vi "Controller Orbit Correction Algorithm.vi"(6 "Resest?":bool, 8 "error in (no error)":errorcluster, 9 "Initial Corrector Kick Vector":dbl[](array[numeric]), 10 "Beam Position Vector":dbl[](array[numeric]), 11 "FOFB Variables":T1) -> (0 "error out":errorcluster, 2 "Corrector Kick Vector":dbl[](array[numeric]), 3 "Good value?":bool=TRUE)   [LabVIEW 2011, in "Controller VIs.lvlib"]
doc: "Computes the correction algorithm to the selected BPM readings and returns the calculated corrector kick vector to be applied to the FOFB actuators."
uses:
  Controller VIs.lvlib
  Types Definitions/Type FOFB Variables.ctl
  Common VIs.lvlib
  Type Definitions.lvlib
panel:
  in  "Maximum allowed disturbance (mm) (1.5)":dbl=1.5 format="%#_6f"
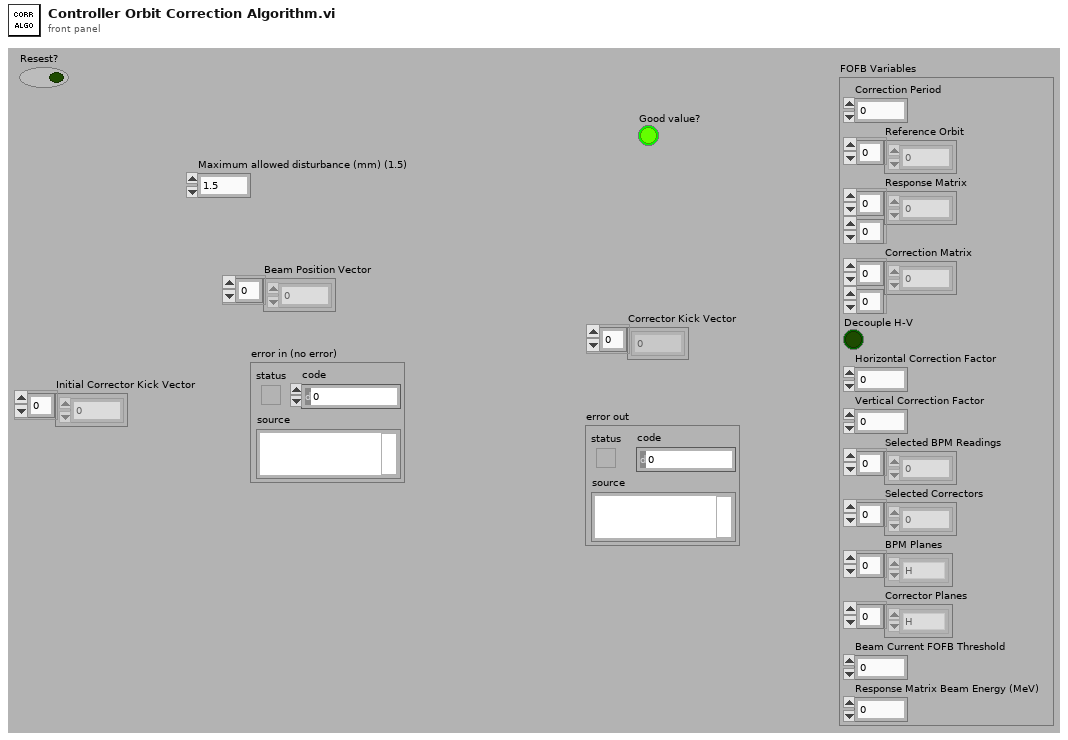
[diagram p1: front panel]
types:
  T1 = typedef "Type Definitions.lvlib/Type FOFB Variables.ctl" = cluster{"Correction Period":u32, "Reference Orbit":dbl[], "Response Matrix":dbl[][], "Correction Matrix":dbl[][], "Decouple H-V":bool, "Horizontal Correction Factor":dbl, "Vertical Correction Factor":dbl, "Selected BPM Readings":u32[], "Selected Correctors":u32[], "BPM Planes":enum8{"H", "V"}[], "Corrector Planes":enum8{"H", "V"}[], "Beam Current FOFB Threshold":dbl, "Response Matrix Beam Energy (MeV)":dbl}
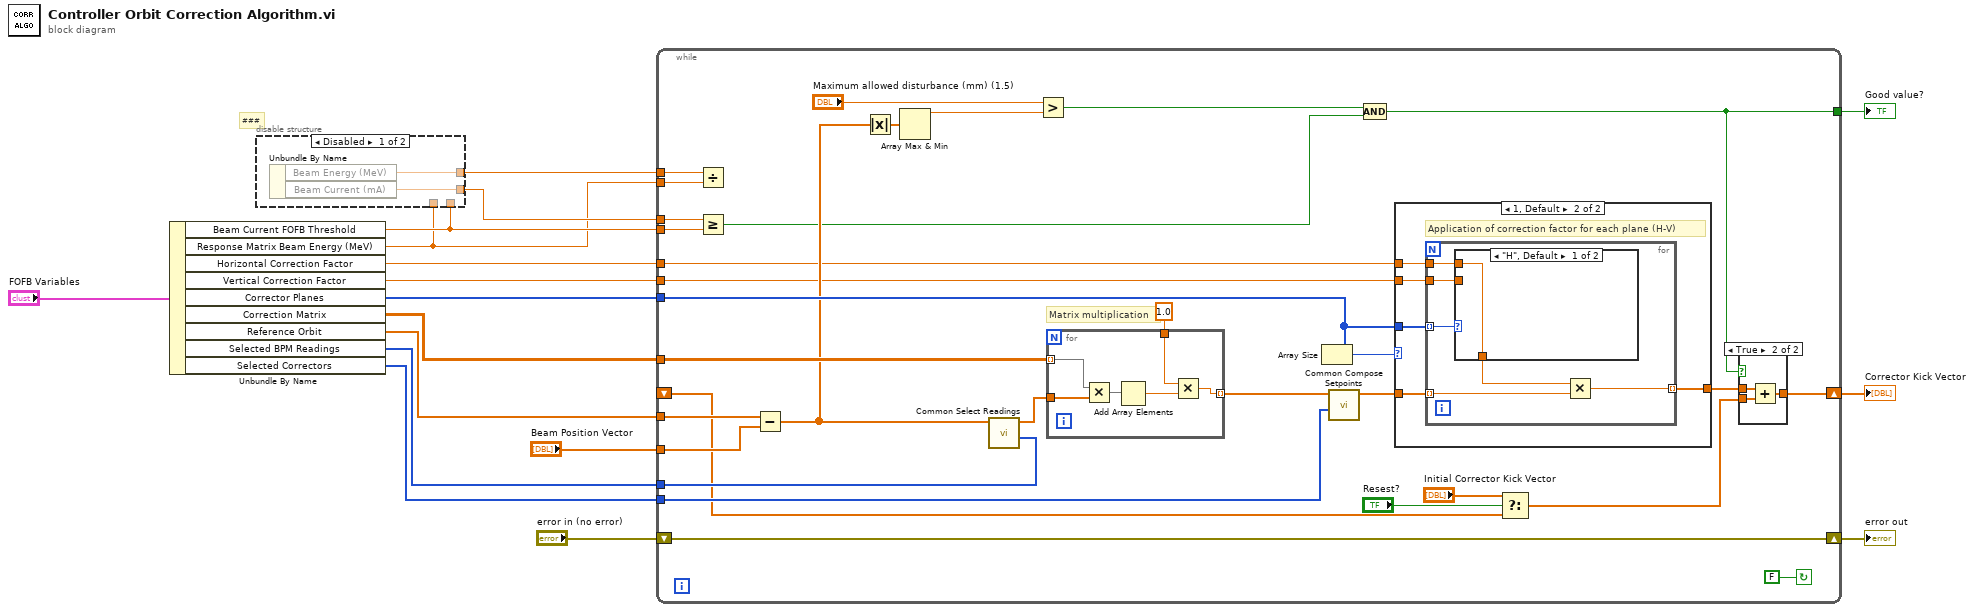
[diagram p0: block diagram]
diagram:
  # "###"
  n1 = Unbundle By Name("FOFB Variables") -> ("Beam Current FOFB Threshold"=w3:dbl, "Response Matrix Beam Energy (MeV)"=w1:dbl, "Horizontal Correction Factor"=w8:dbl, "Vertical Correction Factor"=w7:dbl, "Corrector Planes"=w11:enum8{"H", "V"}[], "Correction Matrix"=w13:dbl[][], "Reference Orbit"=w12:dbl[], "Selected BPM Readings"=w10:u32[], "Selected Correctors"=w9:u32[])
  n2 = disable-structure shown="Disabled" {
    disable-tunnel: [w19 w20] -> w2
    disable-tunnel: [w18 w21] -> w4
    disable-tunnel: w3 -> [_ w21]
    disable-tunnel: w1 -> [_ w20]
    frame Disabled {
      n3 = Unbundle By Name() -> ("Beam Energy (MeV)"=w19:sgl, "Beam Current (mA)"=w18:sgl)  [unwired: 1 in]
    }
    frame Enabled {
    }
  }
  n4 = while {
    tunnel: w13 -> [w53]
    tunnel: w12 -> [w51]
    tunnel: "Beam Position Vector" -> [w50]
    shift-right: [w49] -> w15
    shift-left: "error in (no error)" -> [w49]
    shift-right: [w43] -> w17
    shift-left: _ -> [w42]
    tunnel: w11 -> [w47]
    tunnel: w10 -> [w46]
    tunnel: w9 -> [w45]
    tunnel: w8 -> [w23]
    tunnel: w7 -> [w22]
    tunnel: [w30] -> w6
    tunnel: w4 -> [w29]
    tunnel: w3 -> [w28]
    tunnel: w2 -> [w26]
    tunnel: w1 -> [w25]
    stop <- FALSE continue-if-true
    # "Matrix multiplication"
    n5 = Divide(x=w26, y=w25) -> ()  [unwired: 1 out]
    n6 = Greater Or Equal?(x=w29, y=w28) -> (x >= y?=w27:bool)
    n7 = Subtract(x=w51, y=w50) -> (x-y=w36:dbl[])
    n8 = Absolute Value(x=w36) -> (abs(x)=w35:dbl[])
    n9 = Array Max & Min(array=w35) -> (max value=w33:dbl)  [unwired: 3 out]
    n10 = call "Common Select Readings.vi"("Selected Readings"=w46, "Readings"=w36) -> ("Readings Subset"=w38:dbl[])  [unwired: 9 in]
    n11 = Greater?(x="Maximum allowed disturbance (mm) (1.5)", y=w33) -> (0:w31:bool)
    n12 = for {
      tunnel: w38 -> [w63]
      tunnel: w53 -> [w62] mode=indexing
      tunnel: [w59] -> w39 mode=indexing
      tunnel: 1.0 -> [w58]
      n13 = Multiply(x=w62, y=w63) -> (x*y=w61:dbl[])
      n14 = Add Array Elements(numeric array=w61) -> (sum=w60:dbl)
      n15 = Multiply(x=w58, y=w60) -> (x*y=w59:dbl)
    }
    n16 = Array Size(array=w47) -> (size(s)=w48:i32)
    n17 = call "Common Compose Setpoints.vi"("Selected Correctors"=w45, "Corrector Kicks Subset"=w39) -> ("Corrector Kicks"=w37:dbl[])  [unwired: 9 in]
    n18 = Compound Arithmetic op=AND(w31, w27) -> (w30:bool)
    n19 = case shown="1, Default" w48 {
      tunnel: w37 -> [w64 w69]
      tunnel: [w64 w68] -> w44
      tunnel: w47 -> [_ w67]
      tunnel: w23 -> [_ w66]
      tunnel: w22 -> [_ w65]
      frame 0 {
      }
      frame 1, Default {
        # "Application of correction factor for each plane (H-V)"
        n20 = for {
          tunnel: w69 -> [w74] mode=indexing
          tunnel: [w75] -> w68 mode=indexing
          tunnel: w67 -> [w73] mode=indexing
          tunnel: w66 -> [w71]
          tunnel: w65 -> [w70]
          n21 = case shown="\"H\", Default" w73 {
            tunnel: [w76 w77] -> w72
            tunnel: w71 -> [w76 _]
            tunnel: w70 -> [_ w77]
            frame "H", Default {
            }
            frame "V" {
            }
          }
          n22 = Multiply(x=w72, y=w74) -> (x*y=w75:dbl)
        }
      }
    }
    n23 = Select(t="Initial Corrector Kick Vector", s="Resest?", f=w42) -> (s? t:f=w41:dbl[])
    n24 = case shown="True" w30 {
      tunnel: w44 -> [_ w57]
      tunnel: [w54 w55] -> w43
      tunnel: w41 -> [w54 w56]
      frame False {
      }
      frame True {
        n25 = Add(x=w57, y=w56) -> (x+y=w55:dbl[])
      }
    }
  }
  "error out" <- w15
  "Corrector Kick Vector" <- w17
  "Good value?" <- w6
